vi "Move Down Column.vi"(8 "error in (no error)":errorcluster, 11 "DataGrid Config Dialog in":refnum<class "DataGrid Config Dialog.lvclass">) -> (0 "error out":errorcluster, 3 "DataGrid Config Dialog out":refnum<class "DataGrid Config Dialog.lvclass">)   [LabVIEW 2018, in "DataGrid Config Dialog.lvclass"]
uses:
  DataGrid Config Dialog.lvclass
  DataGrid Config Dialog.lvclass/DataGrid Config Dialog.ctl
  DataGrid Config/Edit Configuration Actions.ctl
  DataGrid Config/DataGrid Config.lvclass
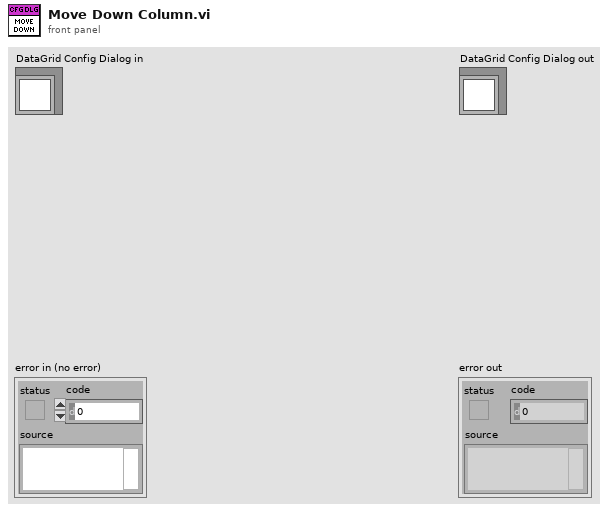
[diagram p1: front panel]
types:
  T1 = typedef "DataGrid Config.lvclass/Edit Configuration Actions.ctl" = enum16{"Add", "Remove", "Update", "Move Up", "Move Down"}
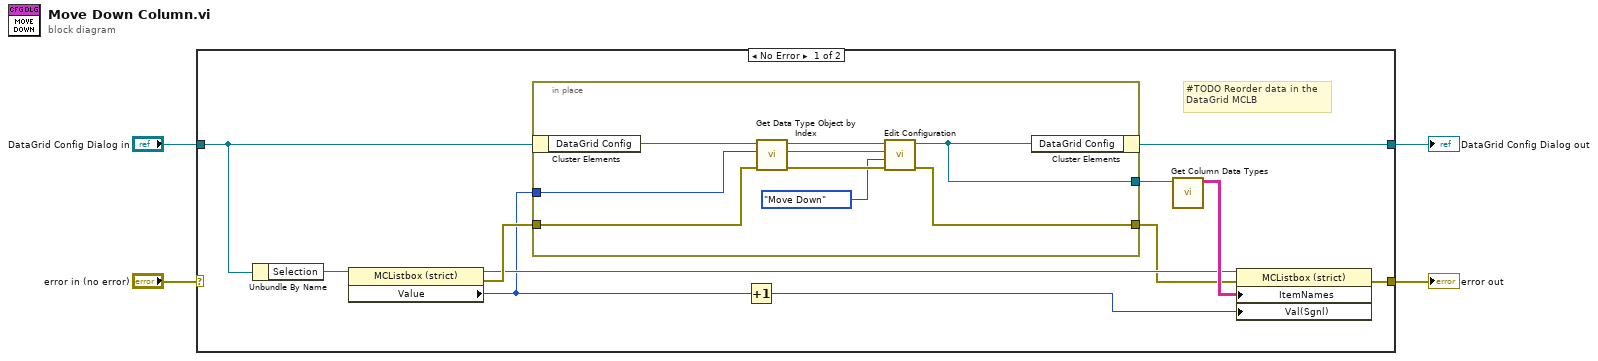
[diagram p0: block diagram]
diagram:
  n1 = case shown="No Error" "error in (no error)" {
    selector: "error in (no error)" -> [_ w26]
    tunnel: [w10 w26] -> w3
    tunnel: [w8 w25] -> w1
    tunnel: "DataGrid Config Dialog in" -> [w15 w25]
    frame No Error {
      # "#TODO Reorder data in the\nDataGrid MCLB"
      n2 = Unbundle By Name(w15) -> ("Selection"=w14:refnum<vi>)
      n3 = property class="MCListbox (strict)"(reference=w14) -> (reference out=w11:refnum<vi>, error out=w13:errorcluster, "Value"=w6:i32)  [unwired: 1 in]
      n4 = in-place {
        in-place-border: w6 -> [w23]
        in-place-border: w13 -> [w18]
        in-place-border: [w16] -> w7
        in-place-border: [w17] -> w9
        n5 = in-place-cluster #1(w15) -> ("DataGrid Config"=w24:refnum<class "DataGrid Config.lvclass">)
        n6 = call "Get Data Type Object by Index.vi"("error in (no error)"=w18, "Index"=w23, "DataGrid Config in"=w24) -> ("error out"=w20:errorcluster, "Data Type Object"=w21:refnum<class "Generic Data Type.lvclass">, "DataGrid Config (dup)"=w22:refnum<class "DataGrid Config.lvclass">)  [unwired: 6 in]
        n7 = call "Edit Configuration.vi"("error in (no error)"=w20, "Edit Configuration Actions"=Edit_Configuration_Actions."Move Down", "Data Type Object"=w21, "DataGrid Config in"=w22) -> ("error out"=w16:errorcluster, "DataGrid Config out"=w17:refnum<class "DataGrid Config.lvclass">)  [unwired: 6 in]
        n8 = in-place-cluster #1("DataGrid Config"=w17) -> (w8:refnum<class "DataGrid Config Dialog.lvclass">)
      }
      n9 = Increment(x=w6) -> (x+1=w5:i32)
      n10 = call "Get Column Data Types.vi"("DataGrid Config"=w9) -> ("Column Data Type Names"=w12:string[][])  [unwired: 10 in]
      n11 = property class="MCListbox (strict)"(reference=w11, error in=w7, "ItemNames"=w12, "Val(Sgnl)"=w5) -> (error out=w10:errorcluster)  [unwired: 1 out]
    }
    frame Error {
    }
  }
  "error out" <- w3
  "DataGrid Config Dialog out" <- w1
